vi "projector validation.vi"(0 "Image Src":T1, 1 "blue channel":T1, 4 "on/off level":dbl, 5 "error in (no error)":errorcluster) -> (16 "on/off":bool, 19 "error out":errorcluster)   [LabVIEW 2019]
uses:
  <vilib>/vision/Image Controls.llb/IMAQ Image.ctl
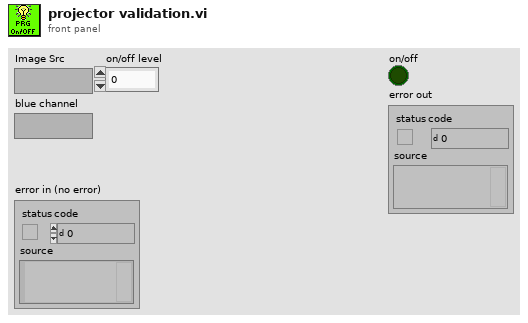
[diagram p1: front panel]
types:
  T1 = typedef "IMAQ Image.ctl" = refnum<image>
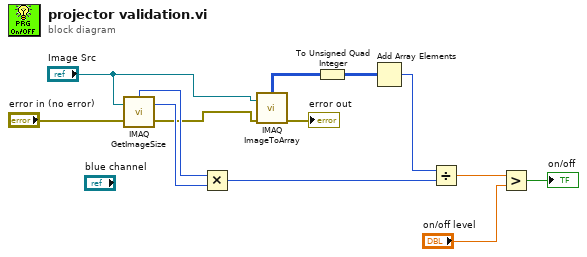
[diagram p0: block diagram]
diagram:
  n1 = call "IMAQ GetImageSize"("Image"="Image Src", "error in (no error)"="error in (no error)") -> ("Y Resolution"=w5:i32, "X Resolution"=w4:i32, "error out"=w1:errorcluster)  [unwired: 2 in]
  n2 = Multiply(x=w4, y=w5) -> (x*y=w10:i32)
  n3 = call "IMAQ ImageToArray"("error in (no error)"=w1, "Image"="Image Src") -> ("error out"=→"error out":errorcluster, "Image Pixels (U8)"=w13:u8[][])  [unwired: 2 in, 3 out]
  n4 = To Unsigned Quad Integer(1:w13) -> (0:w12:u64[][])
  n5 = Add Array Elements(numeric array=w12) -> (sum=w11:u64)
  n6 = Divide(x=w11, y=w10) -> (x/y=w9:dbl)
  n7 = Greater?(x=w9, y="on/off level") -> (0:→"on/off":bool)
